vi "Stereo Logitech Loop.vi"() -> ()   [LabVIEW 2012]
panel:
  out "Blue Flags":cluster{"X Centroid":sgl, "Y Centroid":sgl}[](array[cluster])
  out "Red Flags":cluster{"X Centroid":sgl, "Y Centroid":sgl}[](array[cluster])
  in  "Debug":bool
  in  "stop?":bool caption="Stop (F)"
  out "Gauge":cluster{dbl, dbl}(knob) scale=0.0..50.0
  in  "Left Image":path
  in  "Right Image":path
  out "XY Graph 2":cluster{dbl[], dbl[]}(graph)
  out "XY Graph":cluster{dbl[], dbl[]}(graph)
  out "Right Image":T1(plugin-control)
  out "Left Image":T1(plugin-control)
  in  "Record Button":bool
  in  "Save File Path":path
  out "Time Stamp":timestamp
  out "Image Index":dbl
  out "error out":errorcluster
  in  "error in":errorcluster
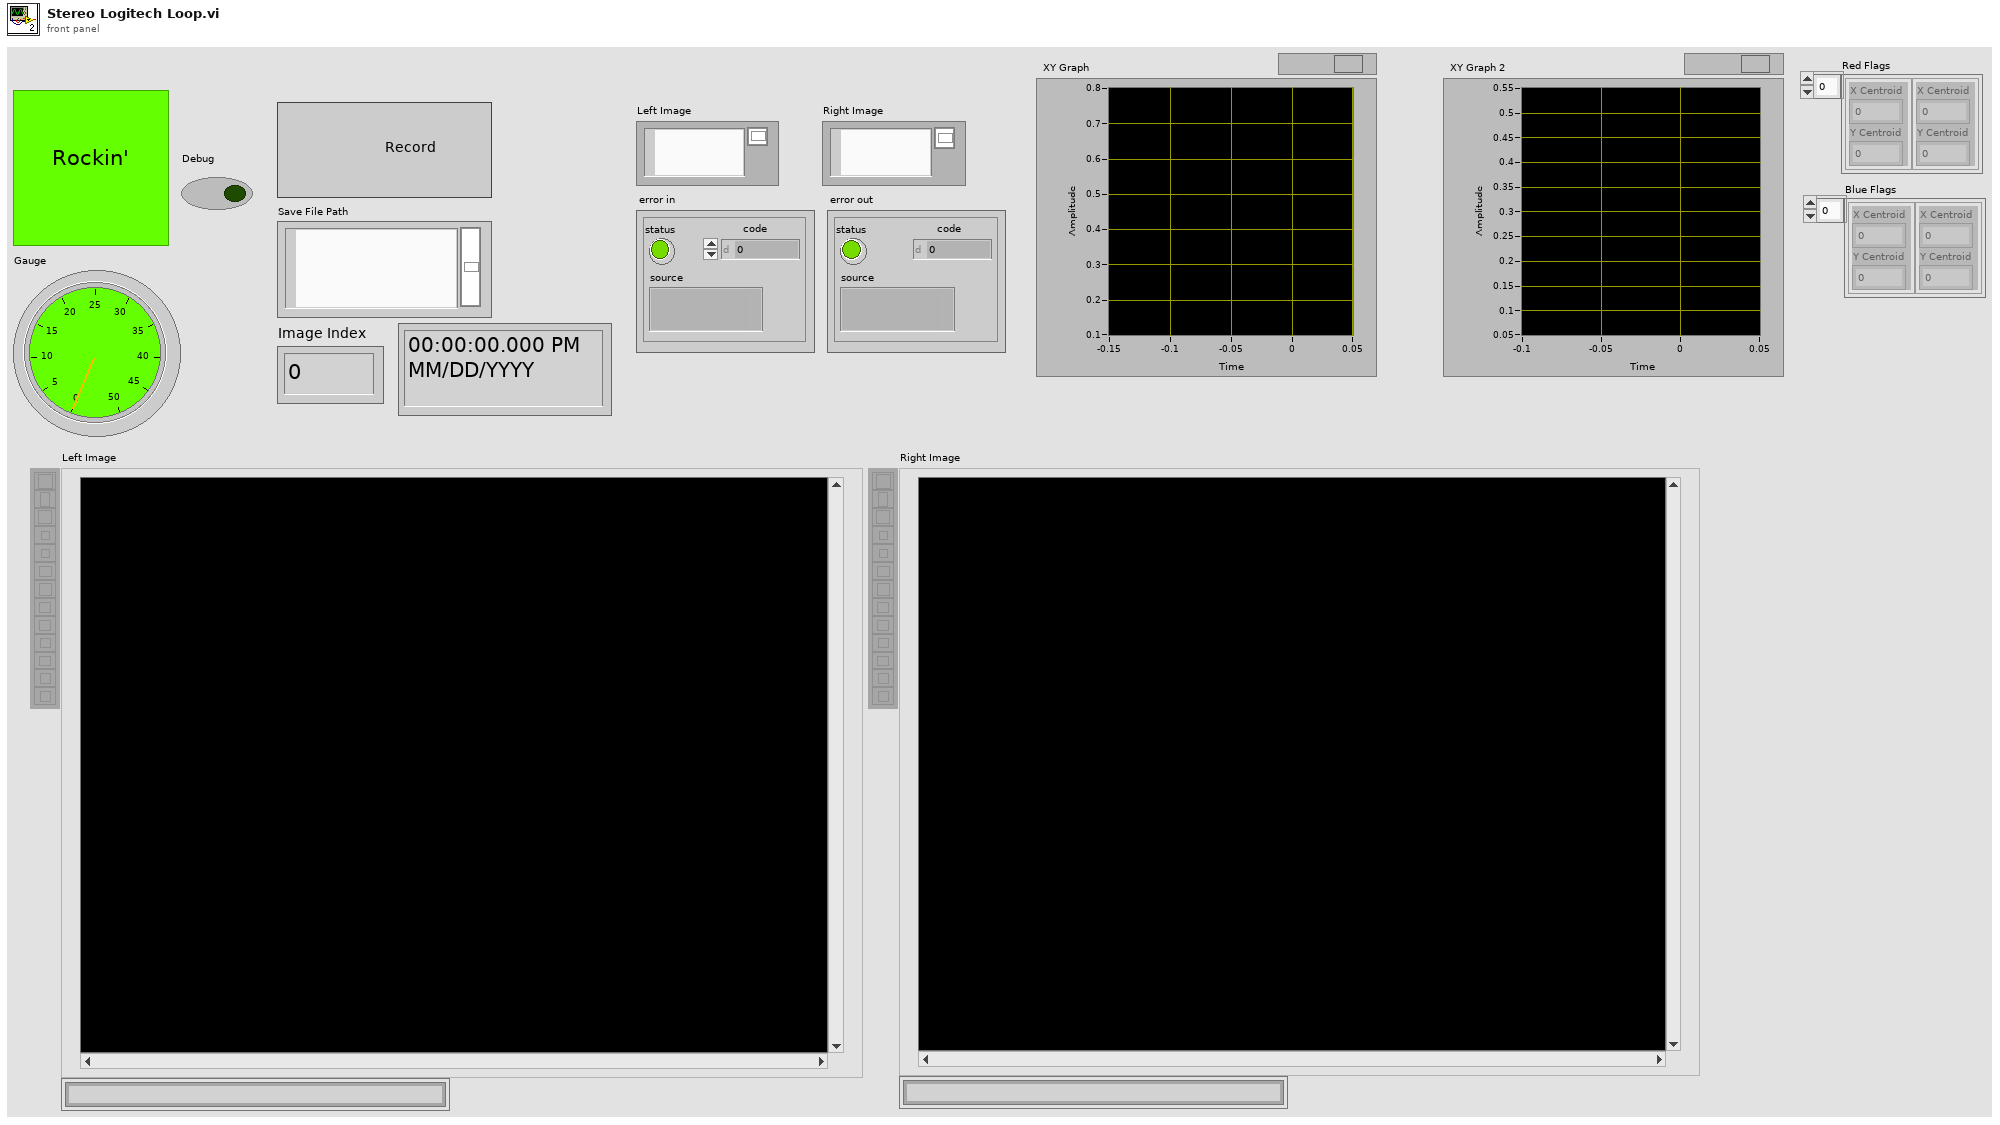
[diagram p1: front panel]
types:
  T1 = typedef "IMAQ Image.ctl" = refnum<image>
  T2 = typedef "Image Type" = u32
  T3 = cluster{"Start Point":cluster{"X":sgl, "Y":sgl}, "End Point":cluster{"X":sgl, "Y":sgl}, "Length":dbl, "Orientation":dbl, "Score":dbl}[]
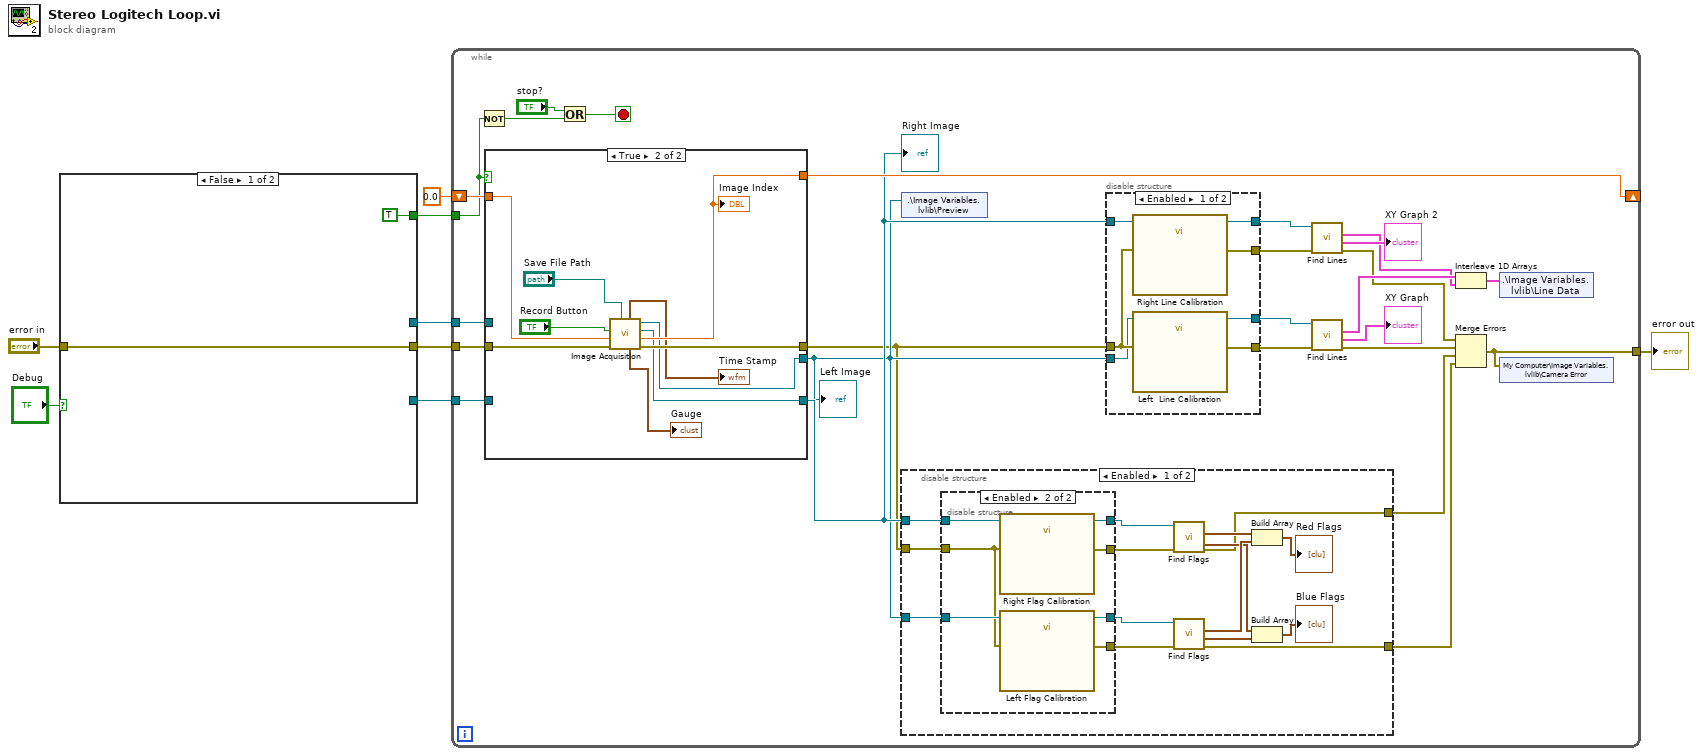
[diagram p0: block diagram]
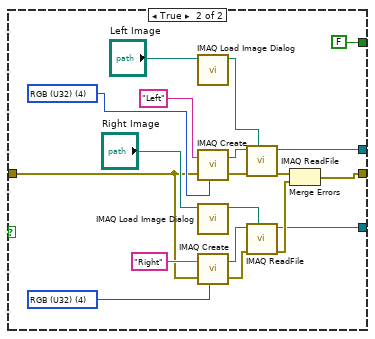
[diagram p6: hidden frame]
diagram:
  n1 = case shown="False" "Debug" {
    tunnel: "error in" -> [w9 w15]
    tunnel: [w9 w14] -> w5
    tunnel: [TRUE FALSE] -> w4
    tunnel: [_ w12] -> w3
    tunnel: [_ w11] -> w2
    frame False {
    }
    frame True {
      w22 = T2 4 items=["Grayscale (U8)", "Grayscale (I16)", "Grayscale (SGL)", "Complex (CSG)", "RGB (U32)", "HSL (U32)", "RGB (U64)", "Grayscale (U16)"] ("Image Type")
      w27 = T2 4 items=["Grayscale (U8)", "Grayscale (I16)", "Grayscale (SGL)", "Complex (CSG)", "RGB (U32)", "HSL (U32)", "RGB (U64)", "Grayscale (U16)"] ("Image Type")
      n2 = call "IMAQ Load Image Dialog"("Start Path"="Left Image") -> ("Path"=w28:path)  [unwired: 8 in, 2 out]
      n3 = call "IMAQ Create"("Image Name"="Left", "Image Type"=w22, "error in (no error)"=w15) -> ("New Image"=w23:T1, "error out"=w24:errorcluster)  [unwired: 2 in]
      n4 = call "IMAQ Load Image Dialog"("Start Path"="Right Image") -> ("Path"=w29:path)  [unwired: 8 in, 2 out]
      n5 = call "IMAQ Create"("Image Name"="Right", "Image Type"=w27, "error in (no error)"=w15) -> ("New Image"=w26:T1, "error out"=w25:errorcluster)  [unwired: 2 in]
      n6 = call "IMAQ ReadFile"("File Path"=w28, "error in (no error)"=w24, "Image"=w23) -> ("error out"=w20:errorcluster, "Image Out"=w11:T1)  [unwired: 4 in, 3 out]
      n7 = call "IMAQ ReadFile"("File Path"=w29, "error in (no error)"=w25, "Image"=w26) -> ("error out"=w21:errorcluster, "Image Out"=w12:T1)  [unwired: 4 in, 3 out]
      n8 = Merge Errors(w20, w21) -> (w14:errorcluster)
    }
  }
  n9 = while {
    tunnel: w5 -> [w55]
    shift-right: [w53] -> _
    shift-left: 0.0 ("Image Index In") -> [w54]
    tunnel: [w37] -> w1
    tunnel: w4 -> [w50]
    tunnel: w3 -> [w52]
    tunnel: w2 -> [w51]
    stop <- w49 stop-if-true
    n10 = Not(x=w50) -> (.not. x?=w48:bool)
    n11 = case shown="True" w50 {
      tunnel: w55 -> [w94 w105]
      tunnel: w54 -> [w95 w104]
      tunnel: [w94 w103] -> w32
      tunnel: [w95 w102] -> w53
      tunnel: [w92 w101] -> w33
      tunnel: [w93 w100] -> w34
      tunnel: w52 -> [w93 _]
      tunnel: w51 -> [w92 _]
      frame False {
      }
      frame True {
        n12 = call "Image Acquisition.vi"("Save File Path"="Save File Path", "Error In"=w105, "Image Index In"=w104, "Record Button"="Record Button") -> ("Error Out"=w103:errorcluster, "Image Index Out"=w102:dbl, "Right Image"=w100:T1, "Left Image"=w101:T1, "Gauge"=→"Gauge":cluster{dbl, dbl}, "Time Stamp"=→"Time Stamp":timestamp)  [unwired: 2 in]
        "Image Index" <- w102
      }
    }
    "Left Image" <- w33
    "Right Image" <- w34
    n13 = Or(x="stop?", y=w48) -> (x .or. y?=w49:bool)
    n14 = shared-variable ".\\Image Variables.lvlib\\Preview"(w33) -> ()  [unwired: 1 in, 1 out]
    n15 = disable-structure shown="Enabled" {
      disable-tunnel: w34 -> [w56 _]
      disable-tunnel: w33 -> [w62 _]
      disable-tunnel: w32 -> [w60 w81]
      disable-tunnel: [w58 w81] -> w31
      disable-tunnel: [w57 w81] -> w30
      frame Enabled {
        n16 = disable-structure shown="Enabled" {
          disable-tunnel: [w73 w76] -> w64
          disable-tunnel: [w72 w79] -> w63
          disable-tunnel: w62 -> [w72 w80]
          disable-tunnel: [w71 w78] -> w61
          disable-tunnel: w60 -> [w71 w74]
          disable-tunnel: [w71 w77] -> w59
          disable-tunnel: w56 -> [w73 w75]
          frame Disabled {
          }
          frame Enabled {
            n17 = call "Right Flag Calibration"("Image In"=w75, "error in"=w74) -> ("Image Out"=w76:T1, "error out"=w77:errorcluster)  [unwired: 24 in]
            n18 = call "Left Flag Calibration"("Image In"=w80, "error in"=w74) -> ("Image Out"=w79:T1, "error out"=w78:errorcluster)  [unwired: 24 in]
          }
        }
        n19 = call "Find Flags.vi"("error in"=w59, "Image In"=w64) -> ("error out"=w58:errorcluster, "Blue Flag"=w67:cluster{"X Centroid":sgl, "Y Centroid":sgl}, "Red Flag"=w70:cluster{"X Centroid":sgl, "Y Centroid":sgl})  [unwired: 6 in, 1 out]
        n20 = call "Find Flags.vi"("error in"=w61, "Image In"=w63) -> ("error out"=w57:errorcluster, "Blue Flag"=w68:cluster{"X Centroid":sgl, "Y Centroid":sgl}, "Red Flag"=w69:cluster{"X Centroid":sgl, "Y Centroid":sgl})  [unwired: 6 in, 1 out]
        n21 = Build Array(w70, w69) -> (→"Red Flags":cluster{"X Centroid":sgl, "Y Centroid":sgl}[])
        n22 = Build Array(w67, w68) -> (→"Blue Flags":cluster{"X Centroid":sgl, "Y Centroid":sgl}[])
      }
      frame Disabled {
      }
    }
    n23 = disable-structure shown="Enabled" {
      disable-tunnel: w32 -> [w88 w89]
      disable-tunnel: w33 -> [w87 w91]
      disable-tunnel: w34 -> [w86 w90]
      disable-tunnel: [w85 w91] -> w43
      disable-tunnel: [w84 w89] -> w42
      disable-tunnel: [w83 w90] -> w41
      disable-tunnel: [w82 w89] -> w40
      frame Enabled {
        n24 = call "Right Line Calibration"("Image In"=w86, "error in"=w88) -> ("Image Out"=w83:T1, "error out"=w82:errorcluster)  [unwired: 24 in]
        n25 = call "Left  Line Calibration"("Image In"=w87, "error in"=w88) -> ("Image Out"=w85:T1, "error out"=w84:errorcluster)  [unwired: 24 in]
      }
      frame Disabled {
      }
    }
    n26 = call "Find Lines.vi"("error in"=w40, "Image In"=w41) -> ("error out"=w36:errorcluster, "XY Graph"=→"XY Graph 2":cluster{dbl[], dbl[]}, "Lines Calibrated (Shape Detection 1)"=w44:T3)  [unwired: 6 in, 1 out]
    n27 = call "Find Lines.vi"("error in"=w42, "Image In"=w43) -> ("error out"=w35:errorcluster, "XY Graph"=→"XY Graph":cluster{dbl[], dbl[]}, "Lines Calibrated (Shape Detection 1)"=w45:T3)  [unwired: 6 in, 1 out]
    n28 = Interleave 1D Arrays(w45, w44) -> (w39:T3)
    n29 = Merge Errors(w36, w35, w31, w30) -> (w37:errorcluster)
    n30 = shared-variable ".\\Image Variables.lvlib\\Line Data"(w39) -> ()  [unwired: 1 in, 1 out]
    n31 = shared-variable "My Computer\\Image Variables.lvlib\\Camera Error"(w37) -> ()  [unwired: 1 in, 1 out]
  }
  "error out" <- w1
